vi "Sequence Stop.vi"(8 "error in (no error)":errorcluster, 11 "MSX-E3701 in":refnum<class "MSX-E3701.lvclass">) -> (0 "error out":errorcluster, 3 "MSX-E3701 out":refnum<class "MSX-E3701.lvclass">)   [LabVIEW 2014, in "MSX-E3701.lvlib" / "MSX-E3701.lvclass"]
doc: "Detiene la adquisición de datos del Sequence."
uses:
  MSX-E3701.lvclass
  MSX-E3701.lvclass/MSX-E3701.ctl
  API/MSX-E3701_dll.lvlib
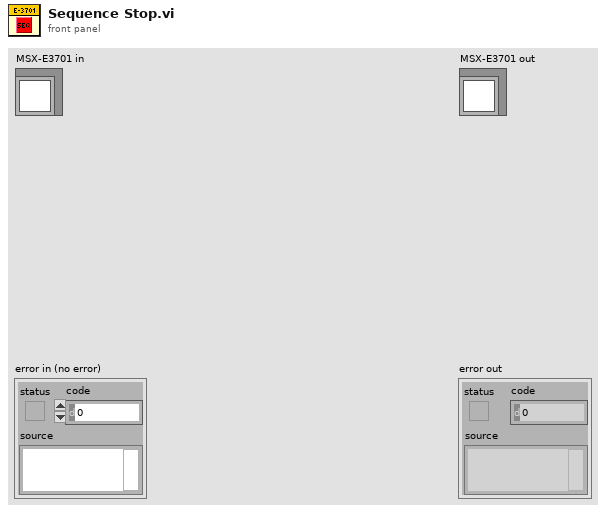
[diagram p1: front panel]
types:
  T1 = typedef "MSX-E3701_dll.lvlib/Connection Data.ctl" = cluster{"MX370x refnum":refnum<k24>, "IP":string, "Connection ID ":refnum<k5>, "MXCommon refnum":refnum<k24>}
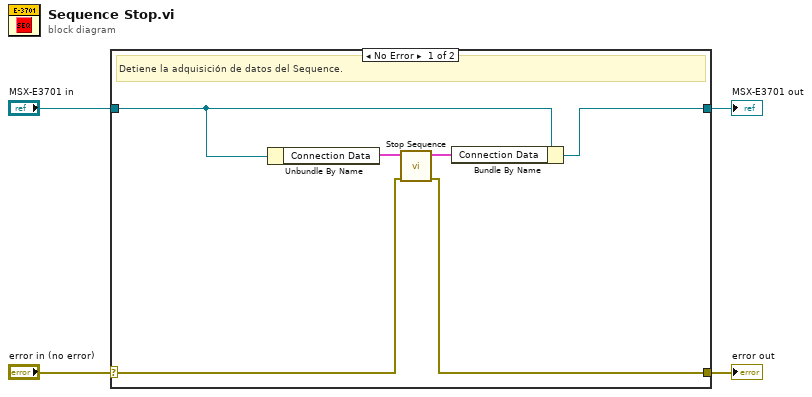
[diagram p0: block diagram]
diagram:
  n1 = case shown="No Error" "error in (no error)" {
    selector: "error in (no error)" -> [w6 w12]
    tunnel: [w5 w12] -> w3
    tunnel: [w9 w11] -> w1
    tunnel: "MSX-E3701 in" -> [w10 w11]
    frame No Error {
      # "Detiene la adquisición de datos del Sequence."
      n2 = Unbundle By Name(w10) -> ("Connection Data"=w7:T1)
      n3 = call "Stop Sequence.vi"("error in (no error)"=w6, "Connection Data In"=w7) -> ("error out"=w5:errorcluster, "Connection Data Out"=w8:T1)  [unwired: 8 in]
      n4 = Bundle By Name(cluster=w10, "Connection Data"=w8) -> (w9:refnum<class "MSX-E3701.lvclass">)
    }
    frame Error {
    }
  }
  "error out" <- w3
  "MSX-E3701 out" <- w1
